vi "Test Create Folder and File.vi"   [LabVIEW 2012]
panel:
  # "见程序框图。"
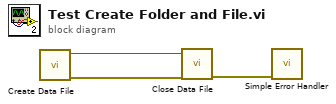
[diagram p0: block diagram]
diagram:
  n1 = call "Create Data File.vi"() -> ("错误输出"=w3:cluster{"状态":bool, "代码":i32, "源":string}, "文件引用句柄"=w1:refnum<file>)  [unwired: 10 in]
  n2 = call "Close Data File.vi"("错误输入"=w3, "文件引用句柄输入"=w1) -> ("错误输出"=w2:errorcluster)  [unwired: 9 in]
  n3 = call <vilib>:"Simple Error Handler.vi"("error in (no error)"=w2) -> ()  [unwired: 4 in, 5 out]
